vi "Sound File Player.vi"(3 "error in (no error)":errorcluster, 4 "Device ID":u32 format="%.0x", 5 "Sound File Path":path=path "sample.wav") -> (0 "error out":errorcluster, 1 "Is Playing?":bool)   [LabVIEW 2013, in "MTA Shift Toolbox.lvlib"]
doc: "This VI illustrates how to play a sound file directly to the speakers. It uses Play Sound File.vi which opens a file and starts playing immediately and asynchronously (as opposed to the method shown in Sound File to Sound Output.vi example)."
uses:
  MTA Shift Toolbox.lvlib
panel:
  in  "stop":bool
  # "This VI plays a sound file directly to your speakers.\n\nInstructions to execute the VI:\n1.  Specify the sound file to read.\n2.  Run the VI. Use the Stop button to stop playback. Otherwise the VI will automatically stop when finished."
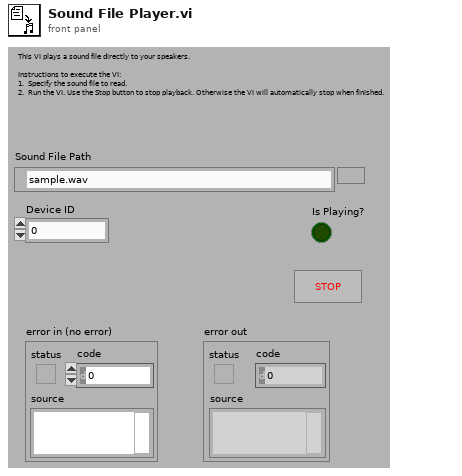
[diagram p1: front panel]
types:
  T1 = typedef "Sound Output Task ID.ctl" = u32
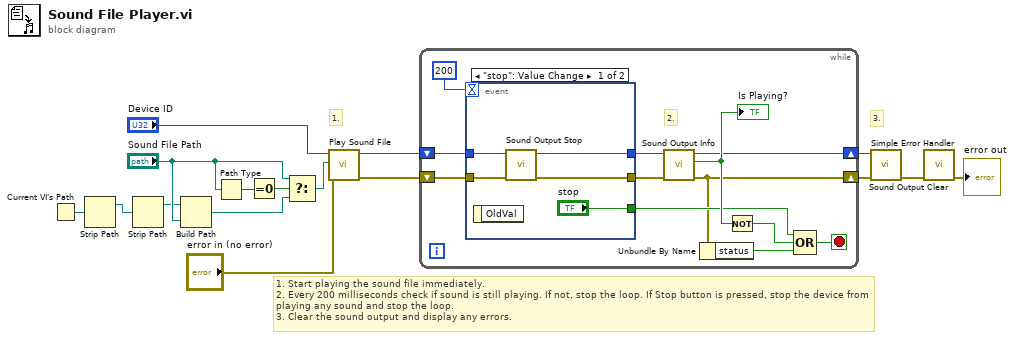
[diagram p0: block diagram]
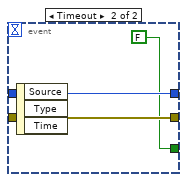
[diagram p2: hidden frame]
diagram:
  # "3."
  # "1."
  # "1. Start playing the sound file immediately.\n2. Every 200 milliseconds check if sound is still playing. If not, stop the loop. If Stop button is pressed, stop the device from playing any sound and stop the loop.\n3. Clear the sound output and display any errors."
  n1 = Current VI's Path() -> (path=w8:path)
  n2 = Strip Path(path=w8) -> (stripped path=w7:path)  [unwired: 1 out]
  n3 = Strip Path(path=w7) -> (stripped path=w6:path)  [unwired: 1 out]
  n4 = Build Path(base path=w6, name or relative path="Sound File Path") -> (appended path=w10:path)
  n5 = Path Type(1:"Sound File Path") -> (0:w12:i16)
  n6 = Equal To 0?(x=w12) -> (x = 0?=w11:bool)
  n7 = Select(t="Sound File Path", s=w11, f=w10) -> (s? t:f=w4:path)
  n8 = call <vilib>:"Play Sound File.vi"("error in (no error)"="error in (no error)", "path"=w4, "device ID"="Device ID") -> ("error out"=w16:errorcluster, "task ID"=w3:T1)  [unwired: 7 in]
  n9 = while {
    shift-right: [w17] -> w15
    shift-left: w16 -> [w26]
    shift-right: [w19] -> w14
    shift-left: w3 -> [w27]
    stop <- w20 stop-if-true
    # "2."
    n10 = event shown="[0] \"stop\": Value Change" {
      selector: _ -> [_ _]
      dyn-events: _ -> [_ _]
      timeout: 200 -> [_ _]
      tunnel: w26 -> [w33 w35]
      tunnel: [w32 w35] -> w25
      tunnel: w27 -> [w31 w36]
      tunnel: [w30 w36] -> w18
      tunnel: ["stop" FALSE ("Stop")] -> w21
      event "stop": Value Change {
        n11 = event-data() -> ()  [unwired: 1 in, 1 out]
        n12 = call <vilib>:"Sound Output Stop.vi"("error in (no error)"=w33, "task ID"=w31) -> ("error out"=w32:errorcluster, "task ID out"=w30:T1)  [unwired: 8 in]
      }
      event Timeout {
        n13 = event-data() -> ()  [unwired: 1 in, 3 out]
      }
    }
    n14 = call <vilib>:"Sound Output Info.vi"("error in (no error)"=w25, "task ID"=w18) -> ("error out"=w17:errorcluster, "is playing?"=w24:bool, "task ID out"=w19:T1)  [unwired: 6 in, 1 out]
    "Is Playing?" <- w24
    n15 = Unbundle By Name(w17) -> ("status"=w23:bool)
    n16 = Not(x=w24) -> (.not. x?=w22:bool)
    n17 = Compound Arithmetic op=OR(w21, w22, w23) -> (w20:bool)
  }
  n18 = call <vilib>:"Sound Output Clear.vi"("error in (no error)"=w15, "task ID"=w14) -> ("error out"=w13:errorcluster)  [unwired: 9 in]
  n19 = call <vilib>:"Simple Error Handler.vi"("error in (no error)"=w13) -> ("error out"=→"error out":errorcluster)  [unwired: 4 in, 4 out]
